vi "AddMergeFile.vi"(8 "error in (no error)":errorcluster, 9 "ExistingFilePath":path, 11 "DataLog in":refnum<class "DataLog.lvclass">) -> (0 "error out":errorcluster, 3 "DataLog out":refnum<class "DataLog.lvclass">)   [LabVIEW 2019, in "DataLog.lvclass"]
uses:
  DataLog.lvclass
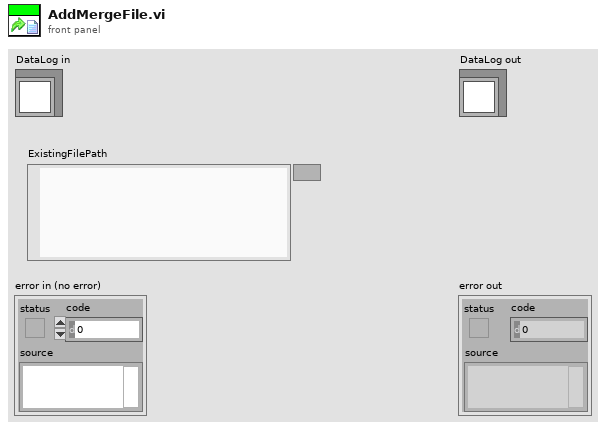
[diagram p1: front panel]
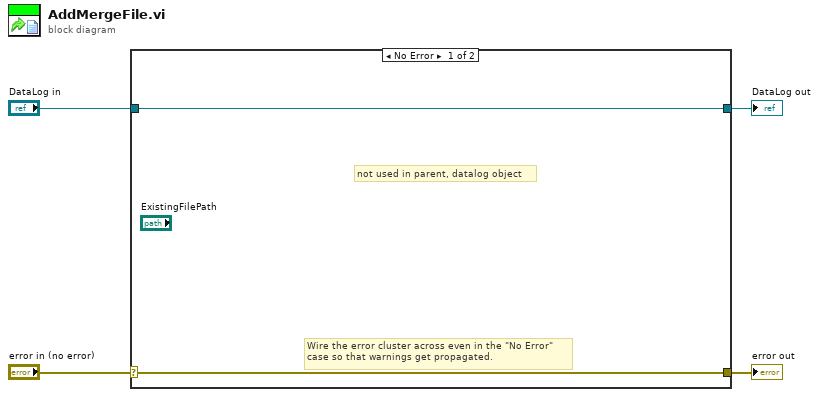
[diagram p0: block diagram]
diagram:
  n1 = case shown="No Error" "error in (no error)" {
    selector: "error in (no error)" -> [w5 w8]
    tunnel: [w5 w8] -> w3
    tunnel: [w6 w7] -> w1
    tunnel: "DataLog in" -> [w6 w7]
    frame No Error {
      # "not used in parent, datalog object"
      # "Wire the error cluster across even in the \"No Error\"\ncase so that warnings get propagated."
    }
    frame Error {
    }
  }
  "error out" <- w3
  "DataLog out" <- w1
